vi "EE300.vi"() -> ()   [LabVIEW 2013]
uses:
  <vilib>/sound2/lvsound2.llb/Sound Data Format.ctl
  <vilib>/sound2/lvsound2.llb/Sampling Mode.ctl
  <vilib>/sound2/lvsound2.llb/Sound File Info (path).vi
  <vilib>/sound2/lvsound2.llb/Sound File Read Open.vi
  <vilib>/sound2/lvsound2.llb/Sound File Read (DBL).vi
  <vilib>/sound2/lvsound2.llb/Sound Output Write (DBL).vi
panel:
  out "B 3":bool
  out "B 2":bool
  out "B1":bool
  out "Amplitude 3":dbl
  out "Amplitude 2":dbl
  out "Amplitude":dbl
  out "detected frequencies":dbl[](array[numeric]) format="%.2p"
  out "Frequency Response":cluster{"f0":dbl, "df":dbl, "magnitude":dbl[]}[](graph)
  out "sound format":T1={"sample rate (S/s)"=22050.0, "number of channels"=2, "bits per sample"=16}
  in  "number of samples/ch (-1: all)":i32=2500
  in  "device ID":u32
  in  "stop":bool
  in  "Volume":dbl(slide)=1.0 scale=0.0..1.0
  in  "Treble":dbl(slide)=1.0 scale=0.0..1.0
  in  "Mid":dbl(slide)=1.0 scale=0.0..1.0
  in  "Bass":dbl(slide)=1.0 scale=0.0..1.0
  in  "path":path=path "C:/Users/ndy102/Desktop/300/Maid_with_the_Flaxen_Hair.wav"
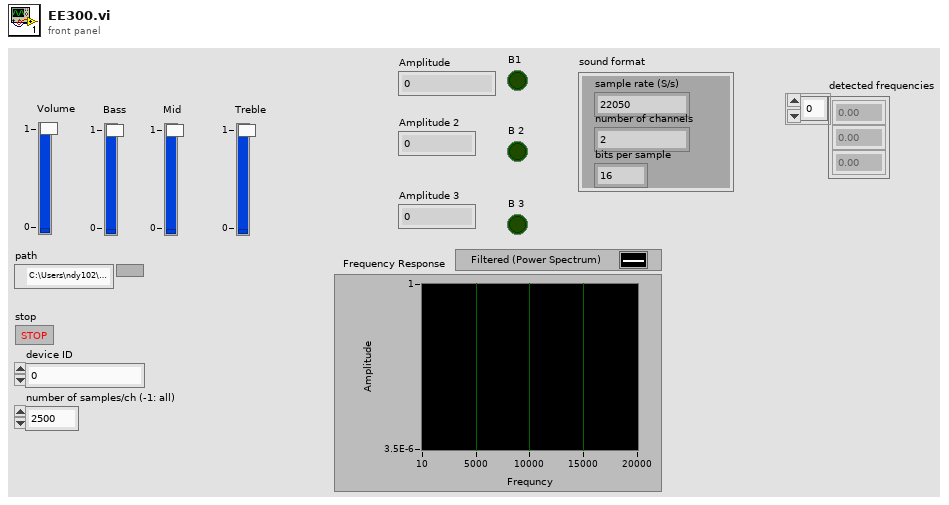
[diagram p1: front panel]
types:
  T1 = typedef "Sound Data Format.ctl" = cluster{"sample rate (S/s)":dbl, "number of channels":i32, "bits per sample":i32}
  T2 = typedef "Sampling Mode.ctl" = i32
  T3 = typedef "Sound File Refnum.ctl" = refnum<file>
  T4 = typedef "Sound Output Task ID.ctl" = u32
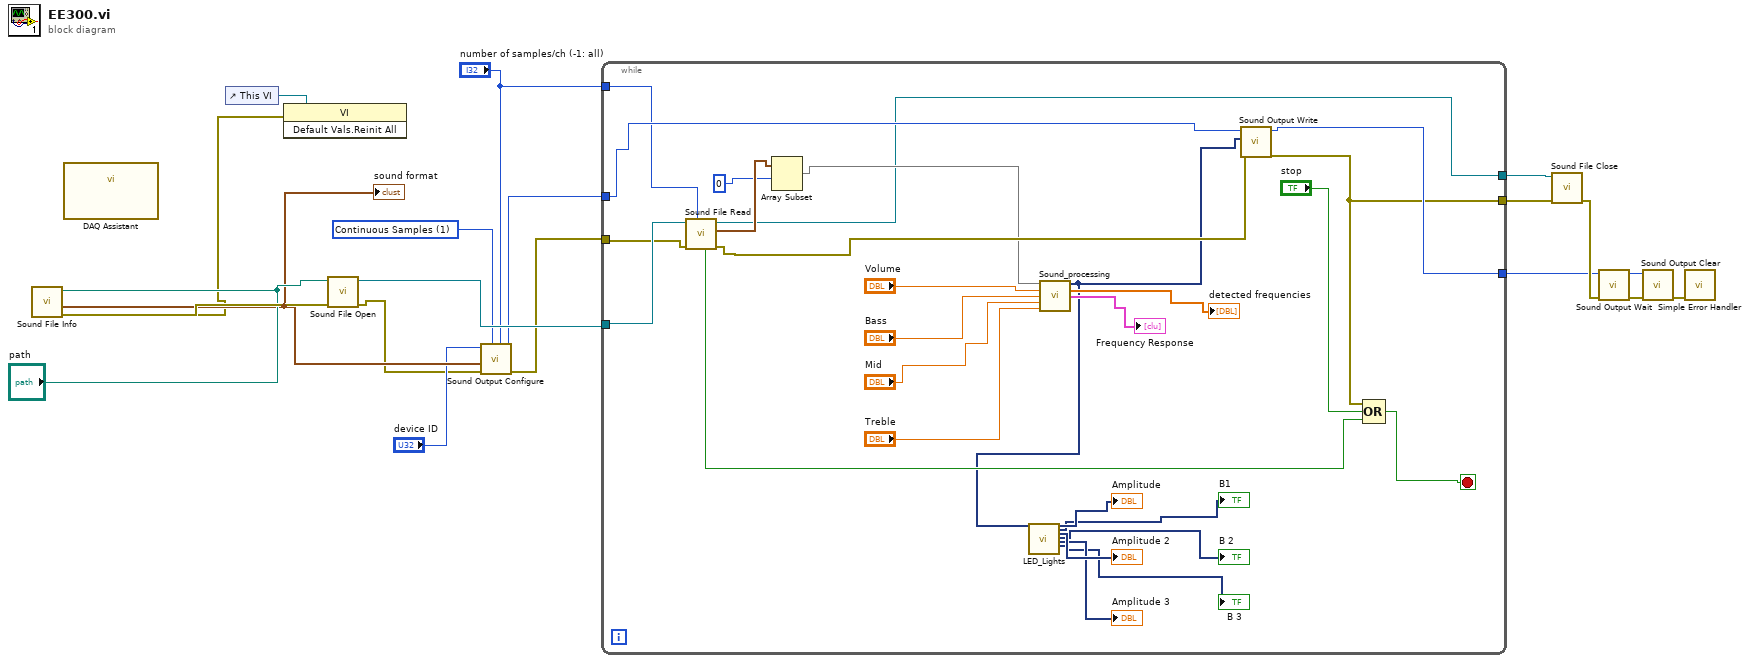
[diagram p0: block diagram]
diagram:
  w6 = T2 1 items=["Finite Samples", "Continuous Samples"] ("sample mode")
  n1 = call "DAQ Assistant"() -> ()  [unwired: 12 in]
  n2 = control-ref of="This VI"() -> (w5:refnum<vi>)
  n3 = invoke class="VI" method="Default Vals.Reinit All"(reference=w5) -> (error out=w4:errorcluster)  [unwired: 2 in, 2 out]
  n4 = call-poly <vilib>:"Sound File Info.vi"("error in (no error)"=w4, "path"="path") -> ("error out"=w19:errorcluster, "sound format"=w17:T1)  [unwired: 6 in, 2 out]
  "sound format" <- w17
  n5 = call-poly <vilib>:"Sound File Open.vi"("error in (no error)"=w19, "path"="path") -> ("error out"=w15:errorcluster, "sound file refnum"=w14:T3)  [unwired: 8 in]
  n6 = call <vilib>:"Sound Output Configure.vi"("number of samples/ch"="number of samples/ch (-1: all)", "sample mode"=w6, "error in (no error)"=w15, "sound format"=w17, "device ID"="device ID") -> ("error out"=w13:errorcluster, "task ID"=w8:T4)  [unwired: 5 in]
  n7 = while {
    tunnel: w14 -> [w46]
    tunnel: w13 -> [w45]
    tunnel: "number of samples/ch (-1: all)" -> [w37]
    tunnel: w8 -> [w40]
    tunnel: [w29] -> w3
    tunnel: [w28] -> w2
    tunnel: [w27] -> w1
    stop <- w41 stop-if-true
    n8 = call-poly <vilib>:"Sound File Read.vi"("number of samples/ch (-1: all)"=w37, "error in (no error)"=w45, "sound file refnum"=w46) -> ("error out"=w44:errorcluster, "data"=w39:waveform(dbl)[], "sound file refnum out"=w27:T3, "end of file?"=w42:bool)  [unwired: 4 in, 1 out]
    n9 = Array Subset(array=w39, index=0) -> (w36:waveform(dbl)[])  [unwired: 1 in]
    n10 = call "Sound_processing.vi"("Array"=w36, "Volume"="Volume", "Bass"="Bass", "Mid"="Mid", "Treble"="Treble") -> ("Dynamic Data"=w26:dynamicdata, "detected frequencies"=→"detected frequencies":dbl[], "Power Spectrum / PSD"=→"Frequency Response":cluster{"f0":dbl, "df":dbl, "magnitude":dbl[]}[])  [unwired: 8 in]
    n11 = call "LED_Lights.vi"("Dynamic Data 4"=w26) -> ("Amplitude"=→"Amplitude":dynamicdata, "Dynamic Data"=→"B1":dynamicdata, "Amplitude 2"=→"Amplitude 2":dynamicdata, "Dynamic Data 2"=→"B 2":dynamicdata, "Amplitude 3"=→"Amplitude 3":dynamicdata, "Dynamic Data 3"=→"B 3":dynamicdata)  [unwired: 21 in]
    n12 = call-poly <vilib>:"Sound Output Write.vi"("error in (no error)"=w44, "data"=w26, "task ID"=w40) -> ("error out"=w28:errorcluster, "task ID out"=w29:T4)  [unwired: 7 in]
    n13 = Compound Arithmetic op=OR(w28, "stop", w42) -> (w41:bool)
  }
  n14 = call <vilib>:"Sound File Close.vi"("error in (no error)"=w2, "sound file refnum"=w1) -> ("error out"=w11:errorcluster)  [unwired: 9 in]
  n15 = call <vilib>:"Sound Output Wait.vi"("error in (no error)"=w11, "task ID"=w3) -> ("error out"=w10:errorcluster, "task ID out"=w12:T4)  [unwired: 8 in]
  n16 = call <vilib>:"Sound Output Clear.vi"("error in (no error)"=w10, "task ID"=w12) -> ("error out"=w9:errorcluster)  [unwired: 9 in]
  n17 = call <vilib>:"Simple Error Handler.vi"("error in (no error)"=w9) -> ()  [unwired: 4 in, 5 out]
